vi "ConvertCodeToArray.vi"(8 "error in (no error)":errorcluster, 11 "baseParser in":refnum<class "baseParser.lvclass">) -> (0 "error out":errorcluster, 3 "baseParser out":refnum<class "baseParser.lvclass">)   [LabVIEW 2013, in "baseParser.lvclass"]
uses:
  baseParser.lvclass
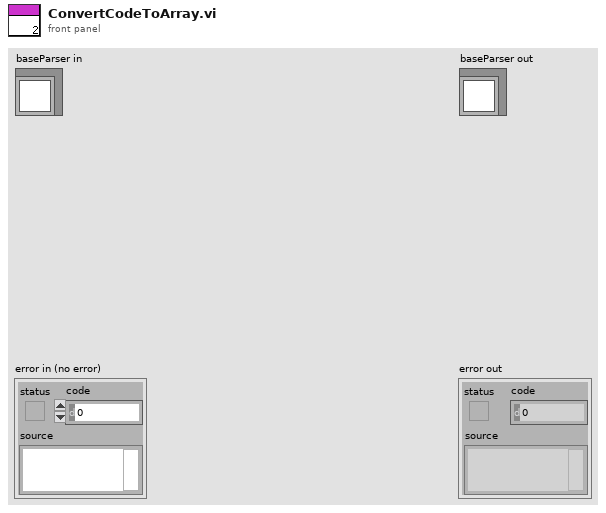
[diagram p1: front panel]
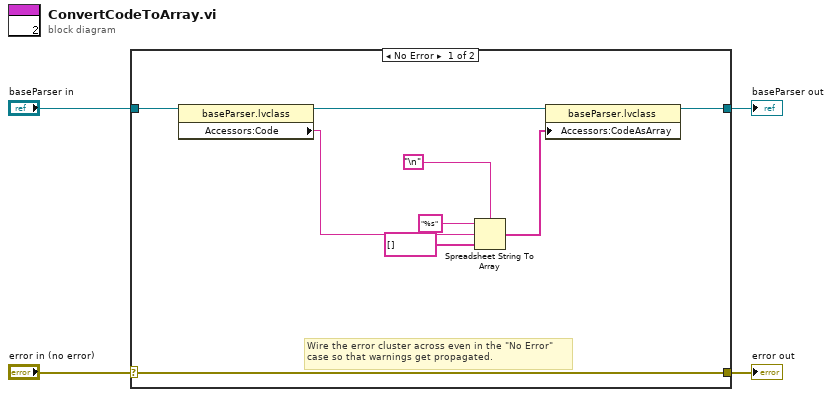
[diagram p0: block diagram]
diagram:
  n1 = case shown="No Error" "error in (no error)" {
    selector: "error in (no error)" -> [w12 w15]
    tunnel: [w12 w15] -> w3
    tunnel: [w6 w14] -> w1
    tunnel: "baseParser in" -> [w13 w14]
    frame No Error {
      # "Wire the error cluster across even in the \"No Error\"\ncase so that warnings get propagated."
      n2 = property class="baseParser.lvclass"(reference=w13) -> (reference out=w11:refnum<class "baseParser.lvclass">, "Accessors:Code"=w7:string)  [unwired: 1 in, 1 out]
      n3 = Spreadsheet String To Array(delimiter (Tab)="\n", format string="%s", spreadsheet string=w7, array type (2D Dbl)=string[] []) -> (array=w5:string[])
      n4 = property class="baseParser.lvclass"(reference=w11, "Accessors:CodeAsArray"=w5) -> (reference out=w6:refnum<class "baseParser.lvclass">)  [unwired: 1 in, 1 out]
    }
    frame Error {
    }
  }
  "error out" <- w3
  "baseParser out" <- w1
